vi "Finish Unflatten VI.vi"(7 "Unflatten Refs":T1, 8 "error in (no error)":errorcluster, 11 "LV-Protoc in":refnum<class "LV-Protoc.lvclass">) -> (0 "error out":errorcluster, 3 "LV-Protoc out":refnum<class "LV-Protoc.lvclass">)   [LabVIEW 2020, in "LV-Protoc.lvlib" / "LV-Protoc.lvclass"]
uses:
  LV-Protoc.lvclass
  Unflatten Refs.ctl
  LV-Protoc.lvlib
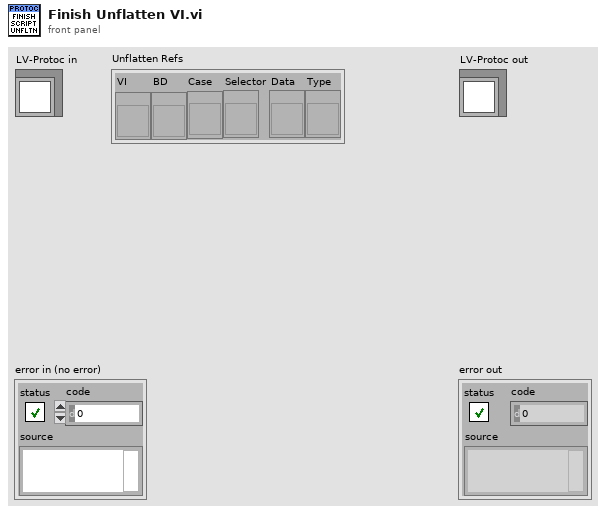
[diagram p1: front panel]
types:
  T1 = typedef "LV-Protoc.lvlib/Unflatten Refs.ctl" = cluster{"VI":refnum<vi>, "BD":refnum<vi>, "Case":refnum<vi>, "Selector":refnum<vi>, "Data":refnum<vi>, "Type":refnum<vi>}
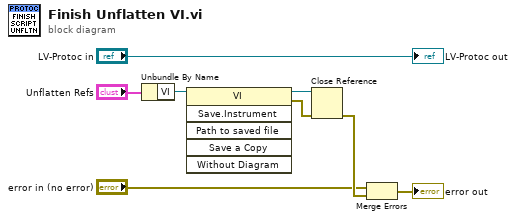
[diagram p0: block diagram]
diagram:
  n1 = Unbundle By Name("Unflatten Refs") -> ("VI"=w7:refnum<vi>)
  n2 = invoke class="VI" method="Save.Instrument"(reference=w7) -> (reference out=w5:refnum<vi>, error out=w6:errorcluster)  [unwired: 5 in, 4 out]
  n3 = Close Reference(reference=w5, error in (no error)=w6) -> (error out=w4:errorcluster)
  n4 = Merge Errors("error in (no error)", w4) -> (→"error out":errorcluster)
  "LV-Protoc out" <- "LV-Protoc in"
